vi "configuration_relative.vi"(7 "project_file":path, 10 "to_relative":bool, 11 "configuration in":T1) -> (3 "configuration out":T1)   [LabVIEW 2015, in "lv-builder-default.lvlib"]
uses:
  lv-builder-default.lvlib
  _controls/configuration.ctl
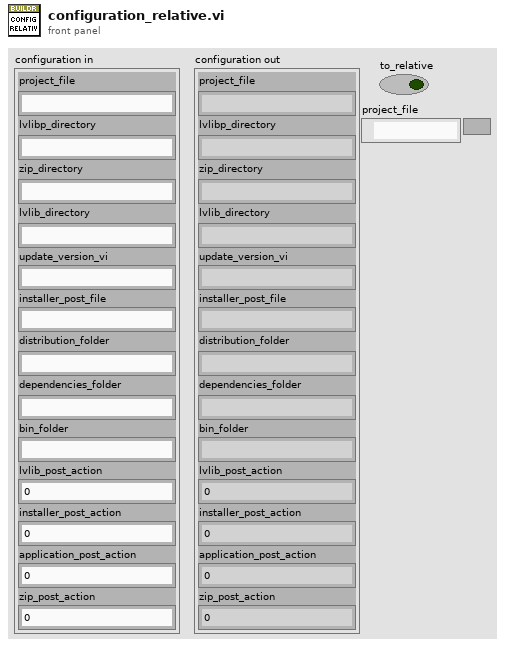
[diagram p1: front panel]
types:
  T1 = typedef "lv-builder-default.lvlib/configuration.ctl" = cluster{"project_file":string, "lvlibp_directory":string, "zip_directory":string, "lvlib_directory":string, "update_version_vi":string, "installer_post_file":string, "distribution_folder":string, "dependencies_folder":string, "bin_folder":string, "lvlib_post_action":u16, "installer_post_action":u16, "application_post_action":u16, "zip_post_action":u16}
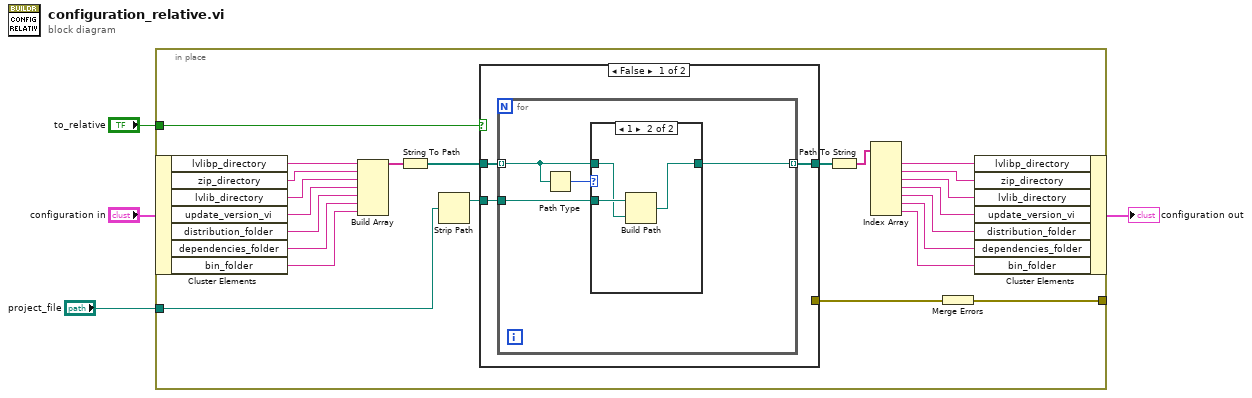
[diagram p0: block diagram]
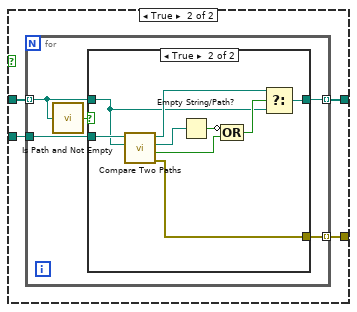
[diagram p3: hidden frame]
diagram:
  n1 = in-place {
    in-place-border: "to_relative" -> [w11]
    in-place-border: [w6] -> _
    in-place-border: "project_file" -> [w5]
    n2 = in-place-cluster #1("configuration in") -> ("lvlibp_directory"=w27:string, "zip_directory"=w26:string, "lvlib_directory"=w25:string, "update_version_vi"=w24:string, "distribution_folder"=w23:string, "dependencies_folder"=w22:string, "bin_folder"=w9:string)
    n3 = Build Array(w27, w26, w25, w24, w23, w22, w9) -> (w21:string[])
    n4 = String To Path(string=w21) -> (path=w20:path[])
    n5 = Strip Path(path=w5) -> (stripped path=w10:path)  [unwired: 1 out]
    n6 = case shown="False" w11 {
      tunnel: w10 -> [w30 w42]
      tunnel: w20 -> [w29 w41]
      tunnel: [w28 w40] -> w19
      tunnel: [_ w39] -> w7
      frame False {
        n7 = for {
          tunnel: w30 -> [w34]
          tunnel: w29 -> [w32] mode=indexing
          tunnel: [w33] -> w28 mode=indexing
          n8 = Path Type(1:w32) -> (0:w31:i16)
          n9 = case shown="1" w31 {
            tunnel: w34 -> [_ w38]
            tunnel: [w35 w37] -> w33
            tunnel: w32 -> [w35 w36]
            frame Default {
            }
            frame 1 {
              n10 = Build Path(base path=w38, name or relative path=w36) -> (appended path=w37:path)
            }
          }
        }
      }
      frame True {
        n11 = for {
          tunnel: w42 -> [w46]
          tunnel: w41 -> [w45] mode=indexing
          tunnel: [w47] -> w40 mode=indexing
          tunnel: [w43] -> w39 mode=indexing
          n12 = call <vilib>:"Is Path and Not Empty.vi"("path"=w45) -> ("Is Path and Not Empty?"=w44:bool)  [unwired: 4 in]
          n13 = case shown="True" w44 {
            tunnel: [w48 w53] -> w47
            tunnel: [_ w52] -> w43
            tunnel: w46 -> [_ w51]
            tunnel: w45 -> [w48 w49]
            frame False {
            }
            frame True {
              n14 = call <vilib>:"Compare Two Paths.vi"("Path 2"=w49, "Path 1"=w51) -> ("error out"=w52:errorcluster, "Path 2 Relative to Path 1?"=w50:bool, "Common Path"=w57:path, "Relative Path from 1 to 2"=w55:path)  [unwired: 6 in]
              n15 = Empty String/Path?(string/path=w57) -> (empty?=w56:bool)
              n16 = Compound Arithmetic op=OR(invert w56, w50) -> (w54:bool)
              n17 = Select(t=w55, s=w54, f=w49) -> (s? t:f=w53:path)
            }
          }
        }
      }
    }
    n18 = Path To String(path=w19) -> (string=w18:string[])
    n19 = Index Array(array=w18) -> (element #1=w17:string, element #2=w16:string, element #3=w15:string, element #4=w14:string, element #5=w13:string, element #6=w12:string, element #7=w8:string)  [unwired: 7 in]
    n20 = Merge Errors(w7) -> (w6:errorcluster)
    n21 = in-place-cluster #1("lvlibp_directory"=w17, "zip_directory"=w16, "lvlib_directory"=w15, "update_version_vi"=w14, "distribution_folder"=w13, "dependencies_folder"=w12, "bin_folder"=w8) -> (→"configuration out":T1)
  }
